vi "InitDemo.vi"(1 "IniFileDir":path, 5 "error in (no error)":errorcluster) -> (15 "SystemEvents.lvclass out":refnum<class "SystemEvents.lvclass">, 19 "error out":errorcluster)   [LabVIEW 2017]
doc: "Singleton wrapper, calls corresponding function in SystemEvents.lvclass."
uses:
  EventHandler/SystemEvents/SystemEvents_class/SystemEvents.lvclass
  EventHandler/SystemEventData/SystemEventsType.ctl
  EventHandler/ActionsOnEvent_class/ActionsOnEvents.lvclass
  <vilib>/Utility/config.llb/Read Key (String).vi
  <vilib>/Utility/config.llb/NI_LVConfig.lvlib
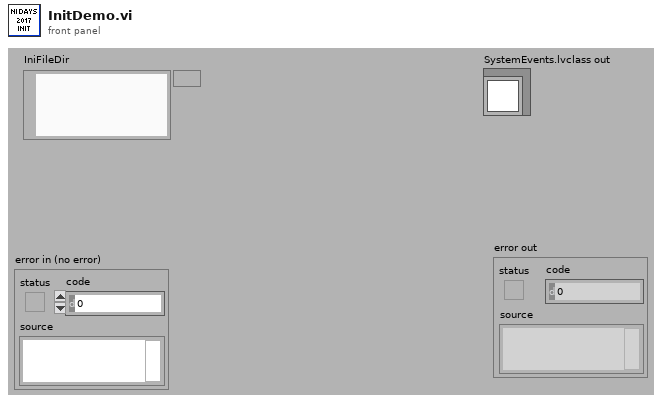
[diagram p1: front panel]
types:
  T1 = typedef "SystemEventsType.ctl" = cluster{"TrigOn":refnum<user-event>, "TrigOff":refnum<user-event>, "Result":refnum<user-event>, "Enable":refnum<user-event>, "Stop":refnum<user-event>, "AnalysisCompleted":refnum<user-event>, "Info":refnum<user-event>}
  T2 = typedef "NI_LVConfig.lvlib/Config Data RefNum.ctl" = refnum<k1>
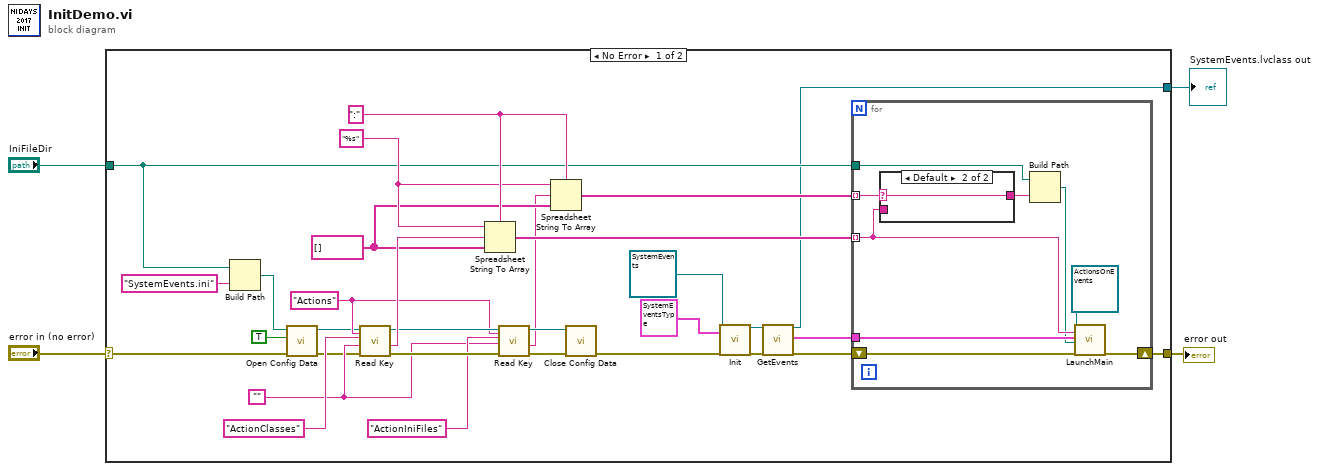
[diagram p0: block diagram]
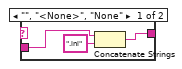
[diagram p2: hidden frame]
diagram:
  n1 = case shown="No Error" "error in (no error)" {
    selector: "error in (no error)" -> [w14 w49]
    tunnel: [w28 w49] -> w3
    tunnel: "IniFileDir" -> [w15 _]
    tunnel: [w5 _] -> w1
    frame No Error {
      w21 = string[] [] ("type (empty)")
      w17 = ""
      w22 = "%s" ("format string")
      w23 = ":" ("delimiter (Tab)")
      w19 = "Actions" ("section")
      n2 = Build Path(base path=w15, name or relative path="SystemEvents.ini") -> (appended path=w11:path)
      n3 = call <vilib>:"Open Config Data.vi"("error in (no error)"=w14, "create file if necessary (T)"=TRUE ("create file if necessary? (F)"), "configuration file path"=w11) -> ("error out"=w13:errorcluster, "refnum"=w10:T2)  [unwired: 6 in, 1 out]
      n4 = call-poly <vilib>:"Read Key.vi"("section"=w19, "error in (no error)"=w13, "default value"=w17, "key"="ActionClasses" ("section"), "refnum"=w10) -> ("error out"=w27:errorcluster, "value"=w33:string, "refnum out"=w25:T2)  [unwired: 3 in, 1 out]
      n5 = Spreadsheet String To Array(delimiter (Tab)=w23, format string=w22, spreadsheet string=w33, array type (2D Dbl)=w21) -> (array=w32:string[])
      n6 = call-poly <vilib>:"Read Key.vi"("section"=w19, "error in (no error)"=w27, "default value"=w17, "key"="ActionIniFiles" ("section"), "refnum"=w25) -> ("error out"=w26:errorcluster, "value"=w20:string, "refnum out"=w24:T2)  [unwired: 3 in, 1 out]
      n7 = Spreadsheet String To Array(delimiter (Tab)=w23, format string=w22, spreadsheet string=w20, array type (2D Dbl)=w21) -> (array=w16:string[])
      n8 = call <vilib>:"Close Config Data.vi"("error in (no error)"=w26, "refnum"=w24) -> ("error out"=w8:errorcluster)  [unwired: 8 in, 1 out]
      n9 = call-dynamic "Init.vi"("SystemEvents in"=refnum<class "SystemEvents.lvclass"> refnum, "Events"=T1 {"TrigOn"=refnum, "TrigOff"=refnum, "Result"=refnum, "Enable"=refnum, "Stop"=refnum, "AnalysisCompleted"=refnum, "Info"=refnum}, "error in (no error)"=w8) -> ("SystemEvents out"=w30:refnum<class "SystemEvents.lvclass">, "error out"=w31:errorcluster)  [unwired: 15 out]
      n10 = call-dynamic "GetEvents.vi"("SystemEvents.lvclass in"=w30, "error in (no error)"=w31) -> ("SystemEvents.lvclass out"=w5:refnum<class "SystemEvents.lvclass">, "Events"=w29:T1, "error out"=w9:errorcluster)  [unwired: 15 out]
      n11 = for {
        shift-right: [w44] -> w28
        shift-left: w9 -> [w41]
        tunnel: w32 -> [w39] mode=indexing
        tunnel: w29 -> [w42]
        tunnel: w16 -> [w40] mode=indexing
        tunnel: w15 -> [w36]
        n12 = case shown="Default" w40 {
          selector: w40 -> [_ w48]
          tunnel: w39 -> [w46 _]
          tunnel: [w45 w48] -> w38
          frame "", "<None>", "None" {
            n13 = Concatenate Strings(w46, ".ini" ("string")) -> (w45:string)
          }
          frame Default {
          }
        }
        n14 = Build Path(base path=w36, name or relative path=w38) -> (appended path=w37:path)
        n15 = call "LaunchMain.vi"("ActionsOnEvents in"=refnum<class "ActionsOnEvents.lvclass"> refnum, "ActionsClass"=w39, "Events"=w42, "IniFile"=w37, "error in (no error)"=w41) -> ("error out"=w44:errorcluster)  [unwired: 14 out]
      }
    }
    frame Error {
    }
  }
  "error out" <- w3
  "SystemEvents.lvclass out" <- w1
